vi "Close.vi"(0 "handle in":T1, 11 "error in (no error)":errorcluster) -> (15 "error out":errorcluster)   [LabVIEW 2017, in "DCAF_JSON_RPC_client.lvlib"]
uses:
  DCAF_JSON_RPC_client.lvlib
  handle.ctl
  <vilib>/httpClient/ClientHandle.ctl
  <vilib>/httpClient/LabVIEWHTTPClient.lvlib
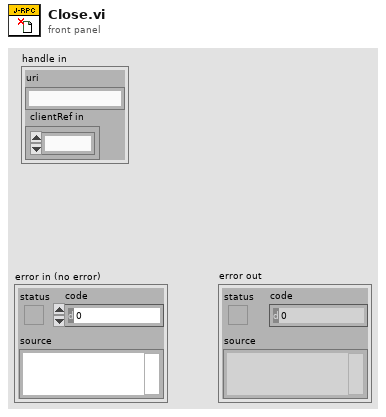
[diagram p1: front panel]
types:
  T1 = typedef "DCAF_JSON_RPC_client.lvlib/handle.ctl" = cluster{"uri":string, " clientRef in":T2}
  T2 = typedef "LabVIEWHTTPClient.lvlib/ClientHandle.ctl" = refnum<k1>
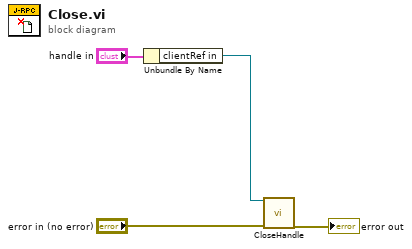
[diagram p0: block diagram]
diagram:
  n1 = Unbundle By Name("handle in") -> ("clientRef in"=w1:T2)
  n2 = call <vilib>:"CloseHandle.vi"("client handle"=w1, "error in (no error)"="error in (no error)") -> ("error out"=→"error out":errorcluster)  [unwired: 13 in]
